vi "Player Info.vi"(11 "Permanent Wall In":refnum<class "Permanent Wall.lvclass">) -> (0 "Defeat Speech":string, 1 "Victory Speech":string, 2 "Name":string, 3 "Permanent Wall Out":refnum<class "Permanent Wall.lvclass">)   [LabVIEW 2015, in "Permanent Wall.lvclass"]
uses:
  Permanent Wall.lvclass
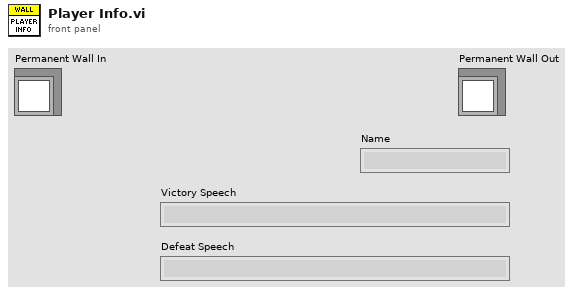
[diagram p1: front panel]
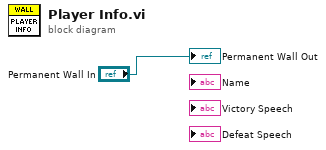
[diagram p0: block diagram]
diagram:
  "Permanent Wall Out" <- "Permanent Wall In"
